vi "Delete Message.vi"(6 "Message ID":string, 8 "error in (no error)":errorcluster, 9 "Pop Receipt":string, 10 "Queue":string, 11 "Azure Session in":refnum<class "Session.lvclass">) -> (0 "error out":errorcluster, 3 "Azure Session out":refnum<class "Session.lvclass">)   [LabVIEW 2015, in "NI_Azure_Queue.lvlib"]
doc: "Deletes a specified message from the queue."
uses:
  NI_Azure_Queue.lvlib
  Core/Session/Session.lvclass
  Core/Name Value Pair.ctl
  Core/Session/Session.lvclass/Session.ctl
  Core/Session/Write HTTP Verb.vi
  Core/Session/Write URL Suffix.vi
  Core/Session/Write Request Parameters.vi
  Core/NI_Azure_Core.lvlib
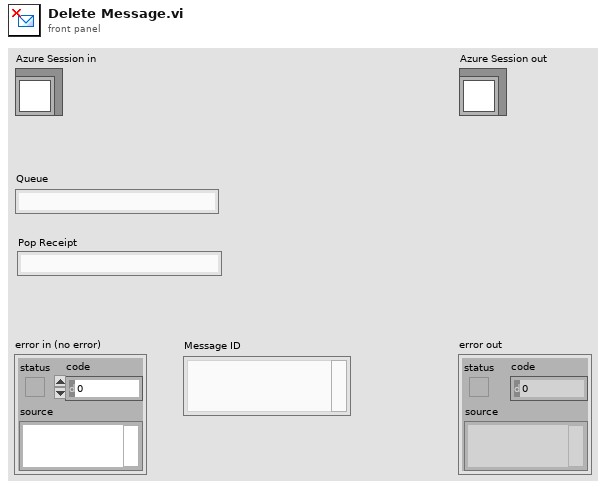
[diagram p1: front panel]
types:
  T1 = typedef "NI_Azure_Core.lvlib/Name Value Pair.ctl" = cluster{"name":string, "value":string}
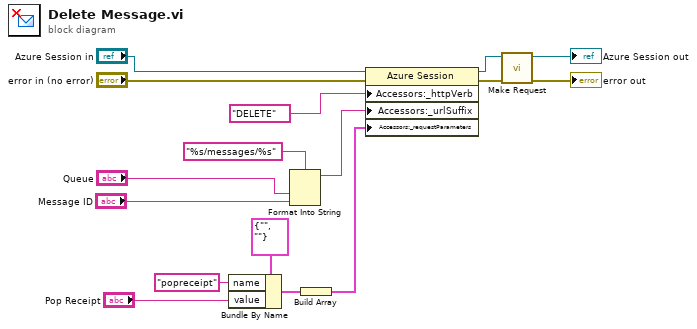
[diagram p0: block diagram]
diagram:
  n1 = Bundle By Name(cluster=T1 {"name"="", "value"=""} ("Name Value Pair"), "name"="popreceipt", "value"="Pop Receipt") -> (w5:T1)
  n2 = Format Into String(format string="%s/messages/%s", "Queue", "Message ID") -> (resulting string=w7:string)  [unwired: 2 in, 1 out]
  n3 = Build Array(w5) -> (w4:T1[])
  n4 = property class="Azure Session"(reference="Azure Session in", error in="error in (no error)", "Accessors:_httpVerb"="DELETE" ("HTTP-Verb"), "Accessors:_urlSuffix"=w7, "Accessors:_requestParameters"=w4) -> (reference out=w9:refnum<class "Session.lvclass">, error out=w11:errorcluster)
  n5 = call "Make Request.vi"("error in (no error)"=w11, "Session in"=w9) -> ("error out"=→"error out":errorcluster, "Session out"=→"Azure Session out":refnum<class "Session.lvclass">)  [unwired: 7 in, 1 out]
